vi "Configure Channels.vi"(8 "error in":errorcluster, 11 "object in":refnum<class "DS1054 Base CFG.lvclass">) -> (0 "error out":errorcluster, 3 "object out":refnum<class "DS1054 Base CFG.lvclass">)   [LabVIEW 2023, in "RIGOL DS1054Z.lvlib" / "DS1054 Base CFG.lvclass"]
uses:
  DS1054 Base CFG.lvclass
  Scope/Scope VISA/Configuration/Scope VISA CFG.lvclass/Scope VISA CFG.ctl
  Configuration Base/Configuration Base.lvclass/Configuration Base.ctl
  13379d92-62cc-4363-acda-c88c807c27a1.vi
  acbb8171-088e-4664-bd13-0f1e166c003a.vi
  0f5d0d8d-dd60-44e3-8a05-a79d933c3f09.vi
  9b939277-0290-4c63-9551-43f1276b4dba.vi
  0b58aace-1cbd-4074-a164-6438e127f828.vi
  b8864795-ac20-4438-a1f8-eecbd4742ffa.vi
  e8d34bdc-91e5-4007-9163-e62f6bb2c44f.vi
  cf25363e-02e6-4a10-b51f-04386fb50273.vi
  fde786d2-5659-4b8b-bdaf-7b854e0c9a4d.vi
  e71cd4f2-48ca-48e1-b9f4-75af4cf58aa5.vi
  <vilib>/JDP Science/JSONtext/Find Item.vi
  <vilib>/JDP Science/JSONtext/Next JSON Value.vi
  <vilib>/JDP Science/JSONtext/String Subset.vi
  <vilib>/JDP Science/JSONtext/Parsing/Advance past next JSON Value (inlined COPY).vi
  <vilib>/JDP Science/JSONtext/Parsing/Advance past whitespace.vi
  <vilib>/JDP Science/JSONtext/Parsing/Advance past String.vi
  <vilib>/JDP Science/JSONtext/Parsing/Advance past Number.vi
  <vilib>/JDP Science/JSONtext/Parsing/Advance past Line Ending.vi
  <vilib>/JDP Science/JSONtext/Parsing/Parse Full Path or Item Name.vi
  <vilib>/JDP Science/JSONtext/Parsing/Advance past Array.vi
  <vilib>/JDP Science/JSONtext/Parsing/Advance past Object.vi
  <vilib>/JDP Science/JSONtext/support/Error Cluster From Code.vi
  <vilib>/JDP Science/JSONtext/Offset/Find Item Locations by Path.vi
  <vilib>/JDP Science/JSONtext/JSON text to Variant.vi
  <vilib>/Utility/error.llb/Error Cluster From Error Code.vi
  <vilib>/JDP Science/JSONtext/LVClass Serializer/JSONtext LVClass Serializer.lvclass
  <vilib>/ErrorRing/Error Ring.xnode
  <instrlib>/RIGOL-DS1054Z-LabVIEW/RIGOL DS1054Z Driver.lvlib
  Scope/Scope VISA/Configuration/Scope VISA CFG.lvclass
  Configuration Base/Configuration Base.lvclass
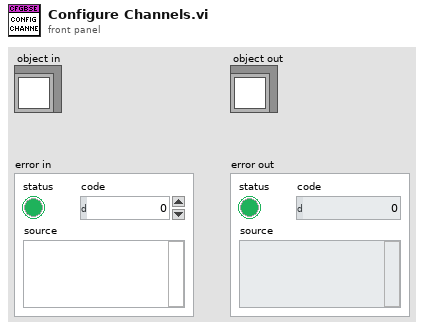
[diagram p1: front panel]
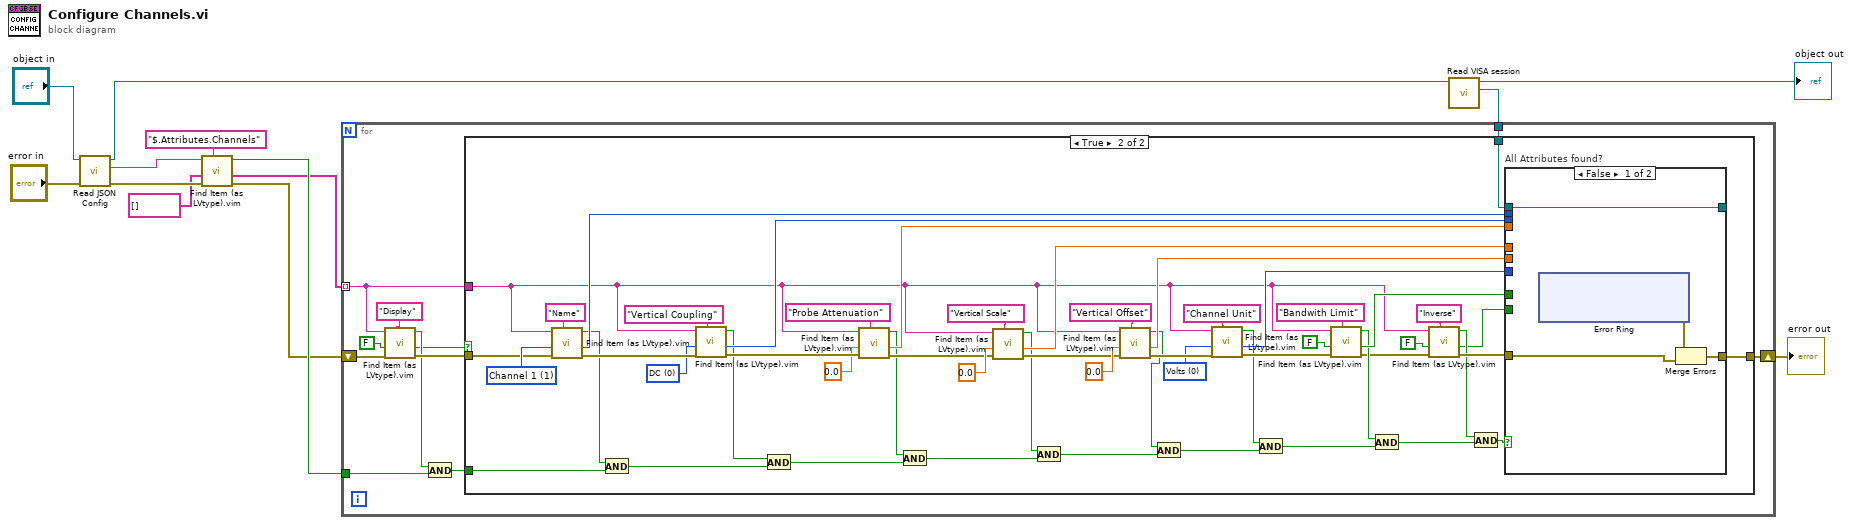
[diagram p0: block diagram]
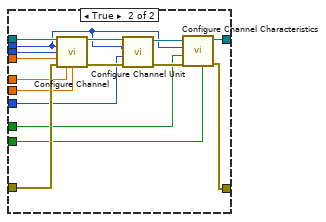
[diagram p3: hidden frame]
diagram:
  n1 = call "Read JSON Config.vi"("error in"="error in", "object in"="object in") -> ("error out"=w8:errorcluster, "<JSON>Config"=w6:string, "object out"=w10:refnum<class "DS1054 Base CFG.lvclass">)  [unwired: 7 in]
  n2 = call "Find Item (as LVtype).vim"("$Path or Item Name"="$.Attributes.Channels", "error in (no error)"=w8, "Data Type and Default Value"=string[] [], "JSON"=w6) -> ("error out"=w5:errorcluster, "Data"=w2:string[], "Found"=w7:bool)  [unwired: 4 in, 1 out]
  n3 = call "Read VISA session.vi"("Scope VISA CFG in"=w10) -> ("VISA session"=w11:refnum<visa-resource-name>, "Scope VISA CFG out"=→"object out":refnum<class "DS1054 Base CFG.lvclass">)  [unwired: 8 in, 1 out]
  n4 = for {
    tunnel: w11 -> [w23]
    tunnel: w7 -> [w22]
    shift-right: [w24] -> w13
    shift-left: w5 -> [w21]
    tunnel: w2 -> [w14] mode=indexing
    n5 = call "Find Item (as LVtype).vim"("$Path or Item Name"="Display", "error in (no error)"=w21, "Data Type and Default Value"=FALSE, "JSON"=w14) -> ("error out"=w20:errorcluster, "Data"=w15:bool, "Found"=w17:bool)  [unwired: 4 in, 1 out]
    n6 = And(x=w17, y=w22) -> (x .and. y?=w18:bool)
    n7 = case shown="True" w15 {
      tunnel: [w25 w78] -> w24
      tunnel: w23 -> [_ w77]
      tunnel: w20 -> [w25 w49]
      tunnel: w18 -> [_ w48]
      tunnel: w14 -> [_ w30]
      frame False {
      }
      frame True {
        w54 = u16 0 items=["DC", "AC", "Ground"] ("Vertical Coupling (0: DC)")
        w55 = u16 1 items=["Channel 1"=1, "Channel 2"=2, "Channel 3"=3, "Channel 4"=4] ("Channel (1: Channel 1)")
        w57 = u16 0 items=["Volts", "Amperes", "Watts", "Unknown"] ("Unit (0: Volts)")
        n8 = call "Find Item (as LVtype).vim"("$Path or Item Name"="Name", "error in (no error)"=w49, "Data Type and Default Value"=w55, "JSON"=w30) -> ("error out"=w75:errorcluster, "Data"=w65:u16, "Found"=w47:bool)  [unwired: 4 in, 1 out]
        n9 = And(x=w47, y=w48) -> (x .and. y?=w45:bool)
        n10 = call "Find Item (as LVtype).vim"("$Path or Item Name"="Vertical Coupling", "error in (no error)"=w75, "Data Type and Default Value"=w54, "JSON"=w30) -> ("error out"=w74:errorcluster, "Data"=w64:u16, "Found"=w46:bool)  [unwired: 4 in, 1 out]
        n11 = And(x=w46, y=w45) -> (x .and. y?=w43:bool)
        n12 = call "Find Item (as LVtype).vim"("$Path or Item Name"="Probe Attenuation", "error in (no error)"=w74, "Data Type and Default Value"=0.0, "JSON"=w30) -> ("error out"=w70:errorcluster, "Data"=w63:dbl, "Found"=w44:bool)  [unwired: 4 in, 1 out]
        n13 = And(x=w44, y=w43) -> (x .and. y?=w41:bool)
        n14 = call "Find Item (as LVtype).vim"("$Path or Item Name"="Vertical Scale", "error in (no error)"=w70, "Data Type and Default Value"=0.0, "JSON"=w30) -> ("error out"=w66:errorcluster, "Data"=w62:dbl, "Found"=w42:bool)  [unwired: 4 in, 1 out]
        n15 = And(x=w42, y=w41) -> (x .and. y?=w39:bool)
        n16 = call "Find Item (as LVtype).vim"("$Path or Item Name"="Vertical Offset", "error in (no error)"=w66, "Data Type and Default Value"=0.0, "JSON"=w30) -> ("error out"=w59:errorcluster, "Data"=w61:dbl, "Found"=w40:bool)  [unwired: 4 in, 1 out]
        n17 = And(x=w40, y=w39) -> (x .and. y?=w37:bool)
        n18 = call "Find Item (as LVtype).vim"("$Path or Item Name"="Channel Unit", "error in (no error)"=w59, "Data Type and Default Value"=w57, "JSON"=w30) -> ("error out"=w58:errorcluster, "Data"=w56:u16, "Found"=w38:bool)  [unwired: 4 in, 1 out]
        n19 = And(x=w38, y=w37) -> (x .and. y?=w35:bool)
        n20 = call "Find Item (as LVtype).vim"("$Path or Item Name"="Bandwith Limit", "error in (no error)"=w58, "Data Type and Default Value"=FALSE, "JSON"=w30) -> ("error out"=w32:errorcluster, "Data"=w50:bool, "Found"=w36:bool)  [unwired: 4 in, 1 out]
        n21 = And(x=w36, y=w35) -> (x .and. y?=w34:bool)
        n22 = call "Find Item (as LVtype).vim"("$Path or Item Name"="Inverse", "error in (no error)"=w32, "Data Type and Default Value"=FALSE, "JSON"=w30) -> ("error out"=w28:errorcluster, "Data"=w26:bool, "Found"=w27:bool)  [unwired: 4 in, 1 out]
        n23 = And(x=w27, y=w34) -> (x .and. y?=w29:bool)
        n24 = case "All Attributes found?" shown="False" w29 {
          tunnel: w77 -> [w81 w103]
          tunnel: w65 -> [_ w91]
          tunnel: w64 -> [_ w96]
          tunnel: w63 -> [_ w95]
          tunnel: w28 -> [w79 w102]
          tunnel: w62 -> [_ w101]
          tunnel: w61 -> [_ w100]
          tunnel: [w80 w90] -> w78
          tunnel: [w81 w92] -> _
          tunnel: w56 -> [_ w97]
          tunnel: w50 -> [_ w89]
          tunnel: w26 -> [_ w88]
          frame False {
            n25 = xnode "Error Ring"() -> ("error out"=w82:errorcluster)
            n26 = Merge Errors(w82, w79) -> (w80:errorcluster)
          }
          frame True {
            n27 = call <instrlib>:"Configure Channel.vi"("VISA resource name"=w103, "Channel (1: Channel 1)"=w91, "Vertical Coupling (0: DC)"=w96, "Probe Attenuation (1.0)"=w95, "error in (no error)"=w102, "Vertical Range (1.0 V)"=w101, "Vertical Offset (0.0 V)"=w100) -> ("VISA resource name out"=w99:refnum<visa-resource-name>, "error out"=w98:errorcluster)  [unwired: 7 in]
            n28 = call <instrlib>:"Configure Channel Unit.vi"("error in (no error)"=w98, "Unit (0: Volts)"=w97, "Channel (1: Channel 1)"=w91, "VISA resource name"=w99) -> ("error out"=w94:errorcluster, "VISA resource name out"=w93:refnum<visa-resource-name>)  [unwired: 6 in]
            n29 = call <instrlib>:"Configure Channel Characteristics.vi"("Invert (F: Disable)"=w88, "error in (no error)"=w94, "BW Limit (F: Disable)"=w89, "Channel (1: Channel 1)"=w91, "VISA resource name"=w93) -> ("error out"=w90:errorcluster, "VISA resource name out"=w92:refnum<visa-resource-name>)  [unwired: 5 in]
          }
        }
      }
    }
  }
  "error out" <- w13
